vi "User Inputs.vi"() -> (3 "Operation States":T2)   [LabVIEW 2014]
uses:
  <vilib>/Rock Robotics/WPI/Solenoid/WPI_SolenoidValue.ctl
  <vilib>/Rock Robotics/WPI/Joystick/WPI_JoystickGetSetRefNum.vi
panel:
  out "Right Axis":dbl
  out "Left Axis":dbl
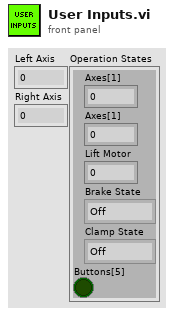
[diagram p1: front panel]
types:
  T1 = typedef "WPI_SolenoidValue.ctl" = enum16{"Off", "On", "Forward", "Reverse"}
  T2 = cluster{"Axes[1]":dbl, "Axes[1]":dbl, "Lift Motor":dbl, "Brake State":T1, "Clamp State":T1, "Buttons[5]":bool}
  T3 = typedef "WPI_JoystickDevRef.ctl" = cluster{"Device":T4}
  T4 = typedef "WPI_JoystickDeviceEnum.ctl" = enum16{"USB 0", "USB 1", "USB 2", "USB 3", "USB 4", "USB 5"}
  T5 = cluster{"Buttons[0]":bool, "Buttons[1]":bool, "Buttons[2]":bool, "Buttons[3]":bool, "Buttons[4]":bool, "Buttons[5]":bool, "Buttons[6]":bool, "Buttons[7]":bool, "Buttons[8]":bool}
  T6 = cluster{"Axes[0]":dbl, "Axes[1]":dbl, "Axes[2]":dbl, "Axes[3]":dbl, "Axes[4]":dbl, "Axes[5]":dbl, "Axes[6]":dbl, "Axes[7]":dbl, "Axes[8]":dbl}
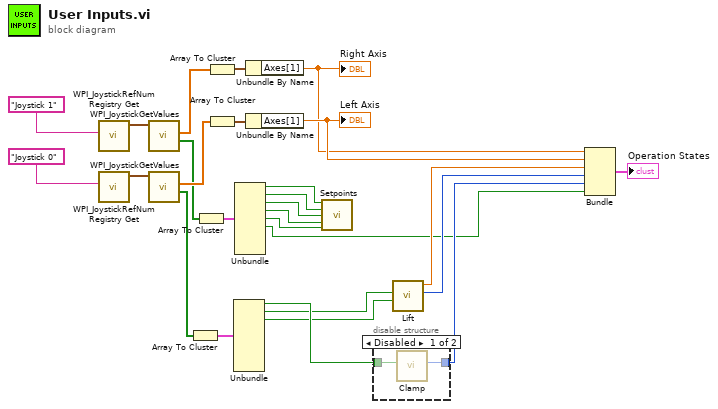
[diagram p0: block diagram]
diagram:
  n1 = call <vilib>:"WPI_JoystickRefNum Registry Get.vi"("refnum name"="Joystick 1") -> ("JoystickDevRef"=w26:T3)  [unwired: 1 in, 9 out]
  n2 = call <vilib>:"WPI_JoystickRefNum Registry Get.vi"("refnum name"="Joystick 0") -> ("JoystickDevRef"=w24:T3)  [unwired: 1 in, 9 out]
  n3 = call <vilib>:"WPI_JoystickGetValues.vi"("JoystickDevRef"=w26) -> ("Buttons"=w8:bool[], "Axes"=w20:dbl[])  [unwired: 6 in, 3 out]
  n4 = call <vilib>:"WPI_JoystickGetValues.vi"("JoystickDevRef"=w24) -> ("Buttons"=w23:bool[], "Axes"=w21:dbl[])  [unwired: 6 in, 3 out]
  n5 = Array To Cluster(array=w23) -> (cluster=w22:T5)
  n6 = Array To Cluster(array=w8) -> (cluster=w9:T5)
  n7 = Array To Cluster(array=w20) -> (cluster=w19:T6)
  n8 = Array To Cluster(array=w21) -> (cluster=w18:T6)
  n9 = Unbundle(w22) -> ("Buttons[0]"=w17:bool, "Buttons[1]"=w13:bool, "Buttons[2]"=w12:bool)  [unwired: 6 out]
  n10 = Unbundle(w9) -> ("Buttons[0]"=w7:bool, "Buttons[1]"=w6:bool, "Buttons[2]"=w5:bool, "Buttons[3]"=w4:bool, "Buttons[4]"=w3:bool, "Buttons[5]"=w2:bool)  [unwired: 3 out]
  n11 = Unbundle By Name(w19) -> ("Axes[1]"=w15:dbl)
  "Right Axis" <- w15
  n12 = Unbundle By Name(w18) -> ("Axes[1]"=w16:dbl)
  "Left Axis" <- w16
  n13 = call "Setpoints.vi"("Button 1"=w7, "Button 2"=w6, "Button 3"=w5, "Button 4"=w4, "Button 5"=w3) -> ()  [unwired: 11 in]
  n14 = disable-structure shown="Disabled" {
    disable-tunnel: w17 -> [w29 _]
    disable-tunnel: [w28 _] -> w11
    frame Disabled {
      n15 = call "Clamp.vi"("Button"=w29) -> ("Clamp State"=w28:T1)  [unwired: 10 in]
    }
    frame Enabled {
    }
  }
  n16 = call "Lift.vi"("Up Button"=w12, "Down Button"=w13) -> ("Brake State"=w10:T1, "Lift Motor"=w14:dbl)  [unwired: 8 in]
  n17 = Bundle("Axes[1]"=w15, "Axes[1]"=w16, "Lift Motor"=w14, "Brake State"=w10, "Clamp State"=w11, "Buttons[5]"=w2) -> (→"Operation States":T2)  [unwired: 1 in]
